vi "P4.vi"() -> ()   [LabVIEW 2019]
panel:
  in  "Stop Button":bool
  out "Boolean":bool
  in  "Número 2":dbl
  in  "Número 1":dbl
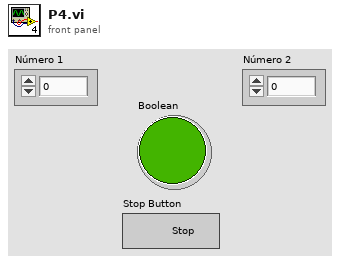
[diagram p1: front panel]
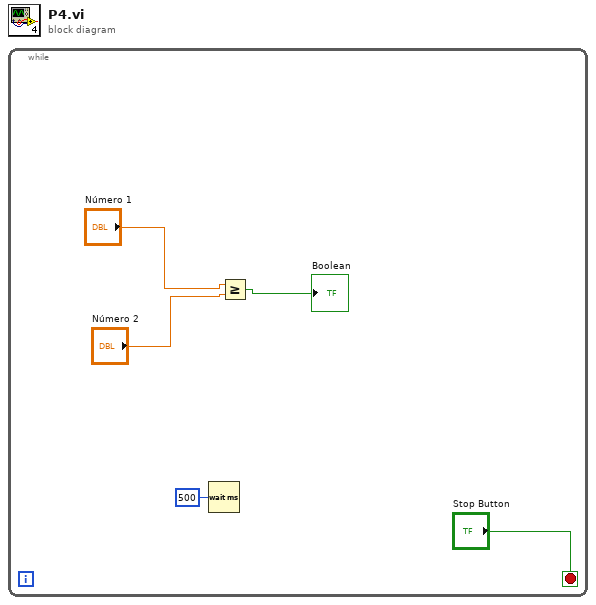
[diagram p0: block diagram]
diagram:
  n1 = while {
    stop <- "Stop Button" stop-if-true
    n2 = Wait (ms)(milliseconds to wait=u32 500) -> ()  [unwired: 1 out]
    n3 = Greater Or Equal?(x="Número 1", y="Número 2") -> (x >= y?=→"Boolean":bool)
  }
